vi "FlatToRichcif_plugincore_Configuration.vi"(5 "OutputClusterType":T1, 11 "InputCluster":T2) -> (3 "OutputCluster":T1)   [LabVIEW 2021, in "CIF_Launcher_server.lvlib"]
uses:
  CIF_Launcher_server.lvlib
  cif_plugincore_Configuration_Flat.ctl
  cif_plugincore_Configuration.ctl
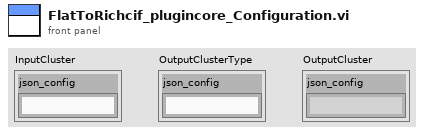
[diagram p1: front panel]
types:
  T1 = typedef "CIF_Launcher_server.lvlib/cif_plugincore_Configuration.ctl" = cluster{"json_config":string}
  T2 = typedef "CIF_Launcher_server.lvlib/cif_plugincore_Configuration_Flat.ctl" = cluster{"json_config":string}
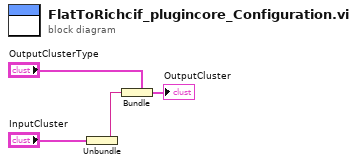
[diagram p0: block diagram]
diagram:
  n1 = Unbundle "Unbundle"("InputCluster") -> ("json_config"=w1:string)
  n2 = Bundle "Bundle"(cluster="OutputClusterType", "json_config"=w1) -> (→"OutputCluster":T1)
